vi "Property Dialog_Setup Show Options.vi"(6 "Properties for Tree In":T1(array[cluster])=[{"Label"="a", "Tag"="a", "Property Type"=enum."Base", "Indent"=0, "Can Read?"=TRUE, "Can Write?"=TRUE, "Is Read?"=FALSE, "Is Write?"=TRUE, "Inactive Parent?"=FALSE, "Unwired?"=FALSE}, {"Label"="b", "Tag"="b", "Property Type"=enum."Scripting", "Indent"=0, "Can Read?"=TRUE, "Can Write?"=FALSE, "Is Read?"=FALSE, "Is Write?"=FALSE, "Inactive Parent?"=FALSE, "Unwired?"=FALSE}, {"Label"="c", "Tag"="c", "Property Type"=enum."Base", "Indent"=0, "Can Read?"=TRUE, "Can Write?"=TRUE, "Is Read?"=FALSE, "Is Write?"=FALSE, "Inactive Parent?"=FALSE, "Unwired?"=FALSE}, {"Label"="d", "Tag"="d", "Property Type"=enum."Private", "Indent"=0, "Can Read?"=TRUE, "Can Write?"=FALSE, "Is Read?"=FALSE, "Is Write?"=FALSE, "Inactive Parent?"=FALSE, "Unwired?"=FALSE}, {"Label"="E", "Tag"="E", "Property Type"=enum."Base", "Indent"=0, "Can Read?"=TRUE, "Can Write?"=TRUE, "Is Read?"=FALSE, "Is Write?"=TRUE, "Inactive Parent?"=FALSE, "Unwired?"=FALSE}, {"Label"="f", "Tag"="f", "Property Type"=enum."Base", "Indent"=0, "Can Read?"=TRUE, "Can Write?"=FALSE, "Is Read?"=FALSE, "Is Write?"=FALSE, "Inactive Parent?"=FALSE, "Unwired?"=FALSE}], 7 "Action":T2, 10 "Select Unwired Ref":refnum<vi>, 11 "Property Disp Cluster":refnum<vi>) -> ()   [LabVIEW 2023]
doc: "Show/hide option booleans for \n\n--Show script/schow private\n--Select unwired termainls (remove items action)"
uses:
  controls/action enum.ctl
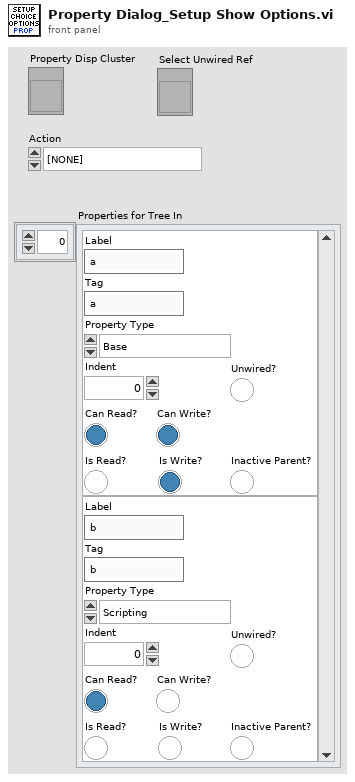
[diagram p1: front panel]
types:
  T1 = cluster{"Label":string, "Tag":string, "Property Type":enum16{"Unknown", "Base", "Scripting", "Private", "Deprecated", "None", "Divider"}, "Indent":u16, "Can Read?":bool, "Can Write?":bool, "Is Read?":bool, "Is Write?":bool, "Inactive Parent?":bool, "Unwired?":bool}[]
  T2 = typedef "action enum.ctl" = enum16{"[NONE]", "APP_SEPARATOR", "Wire Bundle", "Wire Unbundle", "Terminal Unbundle", "Terminal Bundle", "Bundler Move Up", "Bundler Move Down", "Bundler Insert", "Bundler Remove", "Bundler Remove Unwired", "Bundler Reorder", "In Place Insert", "In Place Remove", "In Place Remove Unwired", "In Place Reorder", "Wire Properties", "Wire Method", "Terminal Properties", "Terminal Method", "Property Move Up", "Property Move Down", "Properties Insert", "Properties Remove", "Properties Remove Unwired", "Properties Reorder", "Method Change", "Class For Constant", "Class For Control", "Class For Node", "Class Name to Clipboard"}
  T3 = enum16{"Unknown", "Base", "Scripting", "Private", "Deprecated", "None", "Divider"}
  T4 = cluster{"Show Scripting":bool, "Show Private":bool}
  T5 = enum8{"Enabled", "Disabled", "Disabled and Grayed Out"}
  T6 = enum8{"Enabled", "Disabled", "Disabled and Grayed Out"}[]
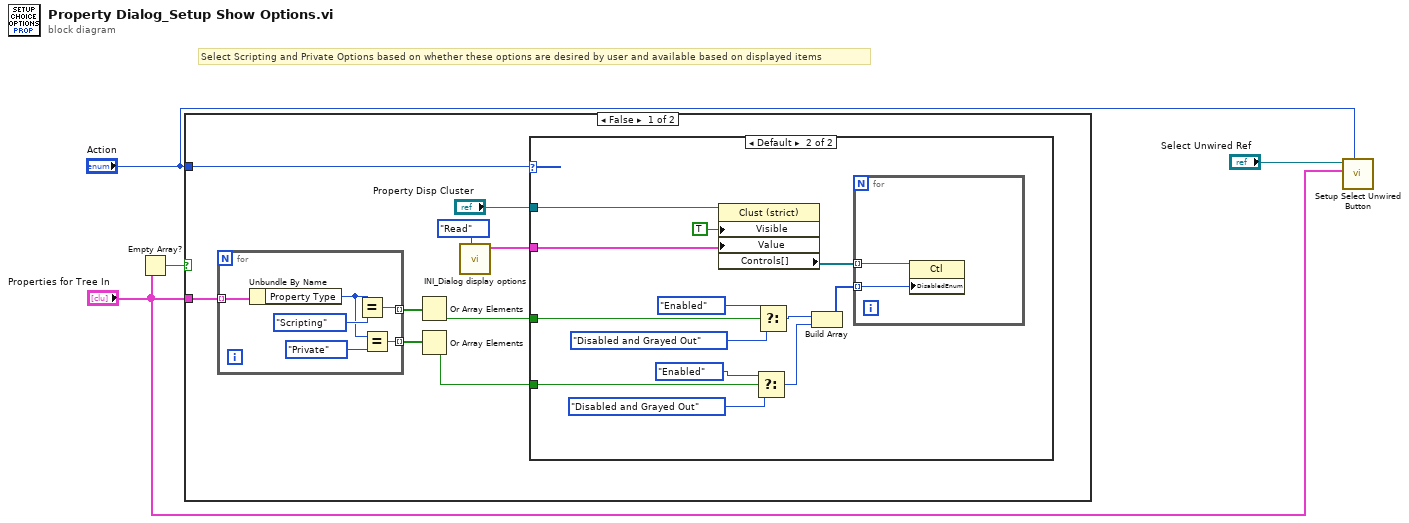
[diagram p0: block diagram]
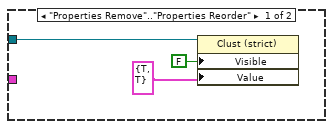
[diagram p2: hidden frame]
diagram:
  # "Select Scripting and Private Options based on whether these options are desired by user and available based on displayed items"
  n1 = Empty Array?(array="Properties for Tree In") -> (empty?=w4:bool)
  n2 = case shown="False" w4 {
    tunnel: "Properties for Tree In" -> [w12 _]
    tunnel: "Action" -> [w7 _]
    frame False {
      n3 = for {
        tunnel: w12 -> [w19] mode=indexing
        tunnel: [w17] -> w11 mode=indexing
        tunnel: [w14] -> w10 mode=indexing
        n4 = Unbundle By Name(w19) -> ("Property Type"=w16:T3)
        n5 = Equal?(x=w16, y=T3."Scripting" ("Property Type")) -> (x = y?=w17:bool)
        n6 = Equal?(x=w16, y=T3."Private" ("Property Type")) -> (x = y?=w14:bool)
      }
      n7 = Or Array Elements(Boolean array=w11) -> (logical OR=w9:bool)
      n8 = Or Array Elements(Boolean array=w10) -> (logical OR=w8:bool)
      n9 = call "INI_Dialog display options.vi"("File Action"=enum16{"Read", "Write"}."Read") -> ("Display Options Out"=w6:T4)  [unwired: 10 in]
      n10 = case shown="Default" w7 {
        tunnel: "Property Disp Cluster" -> [w22 w35]
        tunnel: w6 -> [_ w33]
        tunnel: w9 -> [_ w24]
        tunnel: w8 -> [_ w23]
        frame "Properties Remove".."Properties Reorder" {
          n11 = property class="Clust (strict)"(reference=w22, "Visible"=FALSE, "Value"=T4 {"Show Scripting"=TRUE, "Show Private"=TRUE} ("Show")) -> ()  [unwired: 1 in, 2 out]
        }
        frame Default {
          n12 = property class="Clust (strict)"(reference=w35, "Visible"=TRUE, "Value"=w33) -> ("Controls[]"=w32:refnum<vi>[])  [unwired: 1 in, 2 out]
          n13 = Select(t=T5."Enabled" ("Disabled"), s=w23, f=T5."Disabled and Grayed Out" ("Disabled")) -> (s? t:f=w27:T5)
          n14 = Select(t=T5."Enabled" ("Disabled"), s=w24, f=T5."Disabled and Grayed Out" ("Disabled")) -> (s? t:f=w28:T5)
          n15 = Build Array(w28, w27) -> (w25:T6)
          n16 = for {
            tunnel: w32 -> [w37] mode=indexing
            tunnel: w25 -> [w36] mode=indexing
            n17 = property class="Ctl"(reference=w37, "DisabledEnum"=w36) -> ()  [unwired: 1 in, 2 out]
          }
        }
      }
    }
    frame True {
    }
  }
  n18 = call "Setup Select Unwired Button.vi"("Action"="Action", "Properties for Tree In"="Properties for Tree In", "Boolean in"="Select Unwired Ref") -> ()  [unwired: 8 in, 1 out]
